vi "popUPIngresoODSteelGradeLote.vi"() -> (3 "Listo Ingresar OD SteelGrade Lote":bool=TRUE)   [LabVIEW 2014]
panel:
  in  "ingresarLote":string="numLote"
  in  "ingresarSteelGrade":string="numSteelGrade"
  in  "ingresarOD":string="numeroOD"
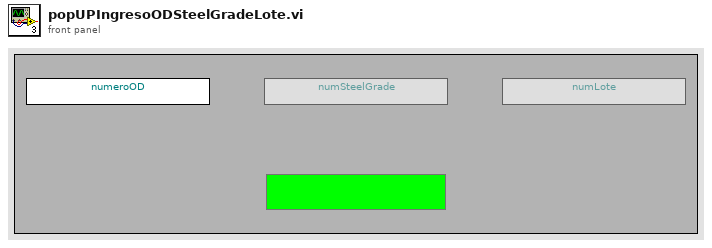
[diagram p1: front panel]
types:
  T1 = enum8{"Enabled", "Disabled", "Disabled and Grayed Out"}
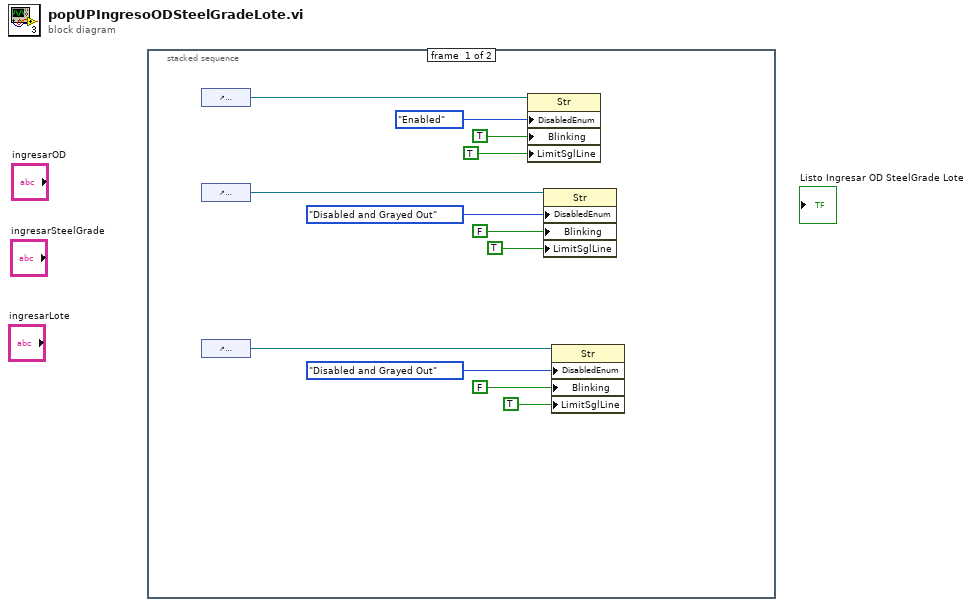
[diagram p0: block diagram]
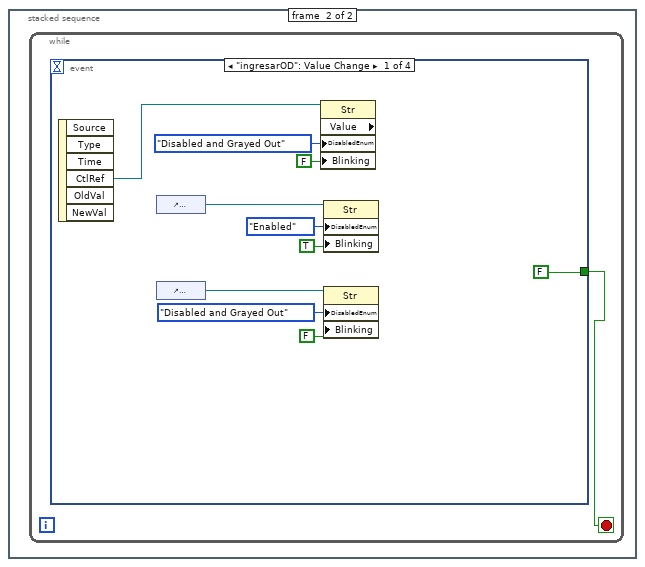
[diagram p2: hidden frame]
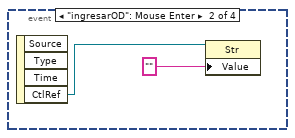
[diagram p3: hidden frame]
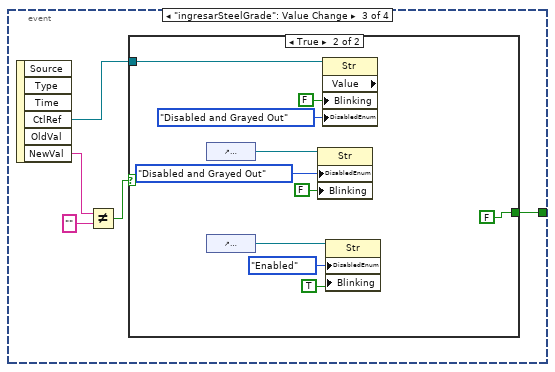
[diagram p4: hidden frame]
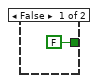
[diagram p5: hidden frame]
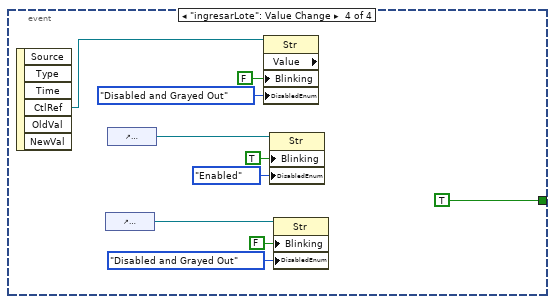
[diagram p6: hidden frame]
diagram:
  n1 = stacked-sequence {
    frame #0 {
      n2 = control-ref of="ingresarOD"() -> (w12:refnum<vi>)
      n3 = control-ref of="ingresarSteelGrade"() -> (w10:refnum<vi>)
      n4 = control-ref of="ingresarLote"() -> (w8:refnum<vi>)
      n5 = property class="Str"(reference=w12, "DisabledEnum"=T1."Enabled" ("Disabled"), "Blinking"=TRUE, "LimitSglLine"=TRUE ("Limit To Single Line?")) -> ()  [unwired: 1 in, 2 out]
      n6 = property class="Str"(reference=w10, "DisabledEnum"=T1."Disabled and Grayed Out" ("Disabled"), "Blinking"=FALSE, "LimitSglLine"=TRUE ("Limit To Single Line?")) -> ()  [unwired: 1 in, 2 out]
      n7 = property class="Str"(reference=w8, "DisabledEnum"=T1."Disabled and Grayed Out" ("Disabled"), "Blinking"=FALSE, "LimitSglLine"=TRUE ("Limit To Single Line?")) -> ()  [unwired: 1 in, 2 out]
    }
    frame #1 {
      n8 = while {
        stop <- w13 stop-if-true
        n9 = event shown="[0] \"ingresarOD\": Value Change" {
          selector: _ -> [_ _ _ _]
          dyn-events: _ -> [_ _ _ _]
          timeout: _ -> [_ _ _ _]
          tunnel: [FALSE _ w29 TRUE] -> w13
          event "ingresarOD": Value Change {
            n10 = event-data() -> ("CtlRef"=w23:refnum<vi>)  [unwired: 1 in, 5 out]
            n11 = control-ref of="ingresarSteelGrade"() -> (w20:refnum<vi>)
            n12 = control-ref of="ingresarLote"() -> (w17:refnum<vi>)
            n13 = property class="Str" props=["Value", "DisabledEnum", "Blinking"](reference=w23, "DisabledEnum"=T1."Disabled and Grayed Out" ("Disabled"), "Blinking"=FALSE) -> ()  [unwired: 1 in, 3 out]
            n14 = property class="Str"(reference=w20, "DisabledEnum"=T1."Enabled" ("Disabled"), "Blinking"=TRUE) -> ()  [unwired: 1 in, 2 out]
            n15 = property class="Str"(reference=w17, "DisabledEnum"=T1."Disabled and Grayed Out" ("Disabled"), "Blinking"=FALSE) -> ()  [unwired: 1 in, 2 out]
          }
          event "ingresarOD": Mouse Enter {
            n16 = event-data() -> ("CtlRef"=w25:refnum<vi>)  [unwired: 1 in, 3 out]
            n17 = property class="Str"(reference=w25, "Value"="") -> ()  [unwired: 1 in, 2 out]
          }
          event "ingresarSteelGrade": Value Change {
            n18 = event-data() -> ("CtlRef"=w30:refnum<vi>, "NewVal"=w28:string)  [unwired: 1 in, 4 out]
            n19 = Not Equal?(x=w28, y="") -> (x != y?=w26:bool)
            n20 = case shown="True" w26 {
              tunnel: w30 -> [_ w41]
              tunnel: [FALSE FALSE] -> w29
              frame False {
              }
              frame True {
                n21 = control-ref of="ingresarOD"() -> (w39:refnum<vi>)
                n22 = control-ref of="ingresarLote"() -> (w36:refnum<vi>)
                n23 = property class="Str"(reference=w39, "DisabledEnum"=T1."Disabled and Grayed Out" ("Disabled"), "Blinking"=FALSE) -> ()  [unwired: 1 in, 2 out]
                n24 = property class="Str" props=["Value", "Blinking", "DisabledEnum"](reference=w41, "Blinking"=FALSE, "DisabledEnum"=T1."Disabled and Grayed Out" ("Disabled")) -> ()  [unwired: 1 in, 3 out]
                n25 = property class="Str"(reference=w36, "DisabledEnum"=T1."Enabled" ("Disabled"), "Blinking"=TRUE) -> ()  [unwired: 1 in, 2 out]
              }
            }
          }
          event "ingresarLote": Value Change {
            n26 = event-data() -> ("CtlRef"=w51:refnum<vi>)  [unwired: 1 in, 5 out]
            n27 = control-ref of="ingresarSteelGrade"() -> (w45:refnum<vi>)
            n28 = control-ref of="ingresarOD"() -> (w48:refnum<vi>)
            n29 = property class="Str" props=["Value", "Blinking", "DisabledEnum"](reference=w51, "Blinking"=FALSE, "DisabledEnum"=T1."Disabled and Grayed Out" ("Disabled")) -> ()  [unwired: 1 in, 3 out]
            n30 = property class="Str"(reference=w48, "Blinking"=TRUE, "DisabledEnum"=T1."Enabled" ("Disabled")) -> ()  [unwired: 1 in, 2 out]
            n31 = property class="Str"(reference=w45, "Blinking"=FALSE, "DisabledEnum"=T1."Disabled and Grayed Out" ("Disabled")) -> ()  [unwired: 1 in, 2 out]
          }
        }
      }
    }
  }
